vi "LoginGui.vi"(11 "Password":string) -> (3 "ok?":bool)   [LabVIEW 2016]
uses:
  LoginGui.Action.ctl
  tools/Config/Config.Global.vi
panel:
  out "_loop":i32(ring)=4
  in  "pwd_Password":string caption="Password"
  in  "CancelButton":bool
  in  "OKButton":bool
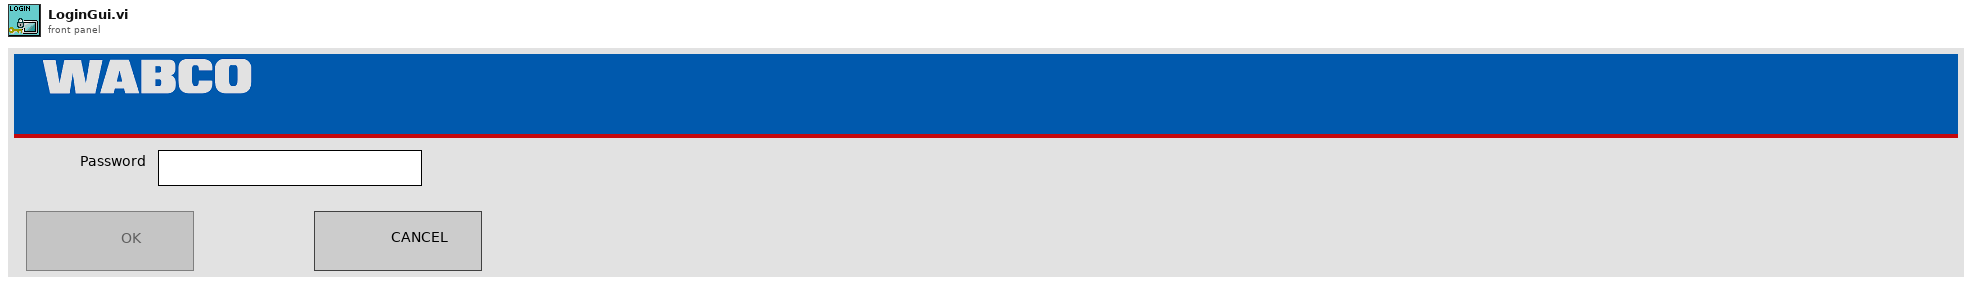
[diagram p1: front panel]
types:
  T1 = typedef "LoginGui.Action.ctl" = enum32{"idle", "constructor", "destructor", "--- Login GUI ---"}
  T2 = enum8{"Enabled", "Disabled", "Disabled and Grayed Out"}
  T3 = enum32{"Invalid", "Default", "Floating", "Floating/Auto-Hide", "Modal"}
  T4 = typedef "FestoCPX.Station.ButtonsState.ctl" = cluster{"Start":bool, "Stop":bool, "Control":bool}
  T5 = typedef "LVPositionTypeDef.ctl" = cluster{"Left":i32, "Top":i32}
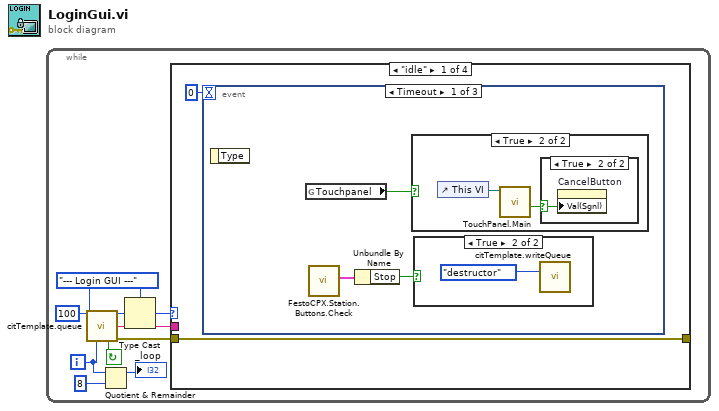
[diagram p0: block diagram]
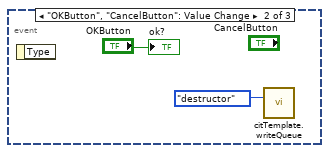
[diagram p5: hidden frame]
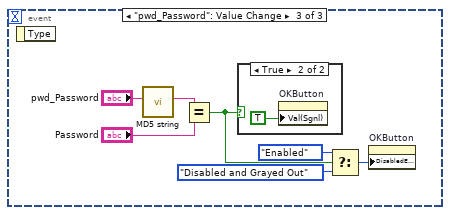
[diagram p6: hidden frame]
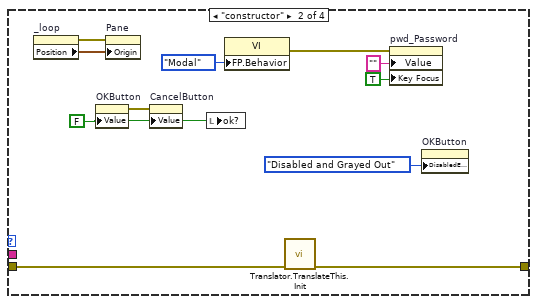
[diagram p8: hidden frame]
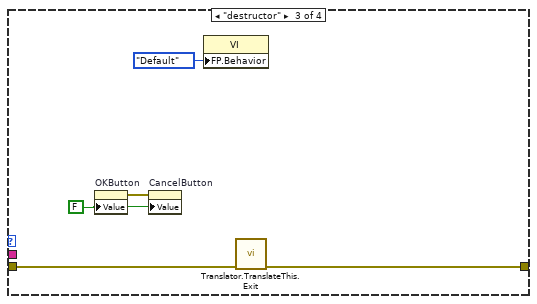
[diagram p9: hidden frame]
diagram:
  n1 = while {
    i -> [w1]
    stop <- w7 continue-if-true
    w6 = LoginGui.Action."--- Login GUI ---" ("Action")
    n2 = call "citTemplate.queue.vi"("ms timeout (250 ms)"=100, "event enum"=w6, "iteration (-1)"=w1) -> ("event out"=w10:u32, "(flatten) data out"=w9:string, "continue"=w7:bool, "error out"=w8:errorcluster)  [unwired: 2 in, 7 out]
    n3 = Quotient & Remainder(x=w1, y=8) -> (x-y*floor(x/y)=→"_loop":i32)  [unwired: 1 out]
    n4 = Type Cast(type=w6, x=w10) -> (*(type *) &x=w5:T1)
    n5 = case shown="\"idle\"" w5 {
      tunnel: w9 -> [_ _ _ _]
      tunnel: w8 -> [w11 w36 w43 w46]
      tunnel: [w11 w35 w42 w46] -> _
      frame "idle" {
        n6 = event shown="[0] Timeout" {
          selector: _ -> [_ _ _]
          dyn-events: _ -> [_ _ _]
          timeout: 0 -> [_ _ _]
          event Timeout {
            n7 = event-data() -> ()  [unwired: 1 in, 1 out]
            n8 = global read "Config.Global.vi" "Touchpanel"() -> (w15:bool)
            n9 = call "FestoCPX.Station.Buttons.Check.vi"() -> ("Buttons.State"=w14:T4)  [unwired: 10 in, 1 out]
            n10 = Unbundle By Name(w14) -> ("Stop"=w13:bool)
            n11 = case shown="True" w15 {
              frame False {
              }
              frame True {
                n12 = control-ref of="This VI"() -> (w18:refnum<vi>)
                n13 = call "TouchPanel.Main.vi"("VI ref"=w18) -> ("Canceled"=w17:bool)  [unwired: 8 in, 2 out]
                n14 = case shown="True" w17 {
                  selector: w17 -> [_ w19]
                  frame False {
                  }
                  frame True {
                    n15 = property on="CancelButton" class="Bool (strict)"("Val(Sgnl)"=w19) -> ()  [unwired: 2 in, 2 out]
                  }
                }
              }
            }
            n16 = case shown="True" w13 {
              frame False {
              }
              frame True {
                n17 = call "citTemplate.writeQueue.vi"("event in (if not connected:all statemachine with data event)"=LoginGui.Action."destructor" ("Action")) -> ()  [unwired: 14 in, 1 out]
              }
            }
          }
          event "OKButton", "CancelButton": Value Change {
            n18 = event-data() -> ()  [unwired: 1 in, 1 out]
            n19 = call "citTemplate.writeQueue.vi"("event in (if not connected:all statemachine with data event)"=LoginGui.Action."destructor" ("Action")) -> ()  [unwired: 14 in, 1 out]
            "ok?" <- "OKButton"
          }
          event "pwd_Password": Value Change {
            n20 = event-data() -> ()  [unwired: 1 in, 1 out]
            n21 = call "MD5 string.vi"("Message String"="pwd_Password") -> ("MD5 message-digest"=w24:string)  [unwired: 10 in]
            n22 = Equal?(x=w24, y="Password") -> (x = y?=w23:bool)
            n23 = case shown="True" w23 {
              frame False {
              }
              frame True {
                n24 = property on="OKButton" class="Bool (strict)"("Val(Sgnl)"=TRUE ("Value (Signaling)")) -> ()  [unwired: 2 in, 2 out]
              }
            }
            n25 = Select(t=T2."Enabled" ("Disabled"), s=w23, f=T2."Disabled and Grayed Out" ("Disabled")) -> (s? t:f=w27:T2)
            n26 = property on="OKButton" class="Bool (strict)"("DisabledEnum"=w27) -> ()  [unwired: 2 in, 2 out]
          }
        }
      }
      frame "constructor" {
        w39 = FALSE ("_b_OK")
        n27 = property on="_loop" class="Ring (strict)"() -> (error out=w37:errorcluster, "Position"=w38:T5)  [unwired: 2 in, 1 out]
        n28 = property on="OKButton" class="Bool (strict)"("Value"=w39) -> (error out=w40:errorcluster)  [unwired: 2 in, 1 out]
        n29 = property on="Pane" class="Pane"(error in=w37, "Origin"=w38) -> ()  [unwired: 1 in, 2 out]
        n30 = property on="CancelButton" class="Bool (strict)"(error in=w40, "Value"=w39) -> ()  [unwired: 1 in, 2 out]
        n31 = local write "ok?"(w39) -> ()
        n32 = property class="VI"("FP.Behavior"=T3."Modal" ("Front Panel Window:Behavior")) -> (error out=w31:errorcluster)  [unwired: 2 in, 1 out]
        n33 = call "Translator.TranslateThis.Init.vi"("error in"=w36) -> ("error out"=w35:errorcluster)  [unwired: 10 in]
        n34 = property on="pwd_Password" class="Str"(error in=w31, "Value"="" ("Password"), "Key Focus"=TRUE) -> ()  [unwired: 1 in, 2 out]
        n35 = property on="OKButton" class="Bool (strict)"("DisabledEnum"=T2."Disabled and Grayed Out" ("Disabled")) -> ()  [unwired: 2 in, 2 out]
      }
      frame "destructor" {
        w44 = FALSE ("_b_OK")
        n36 = property on="OKButton" class="Bool (strict)"("Value"=w44) -> (error out=w45:errorcluster)  [unwired: 2 in, 1 out]
        n37 = property on="CancelButton" class="Bool (strict)"(error in=w45, "Value"=w44) -> ()  [unwired: 1 in, 2 out]
        n38 = property class="VI"("FP.Behavior"=T3."Default" ("Front Panel Window:Behavior")) -> ()  [unwired: 2 in, 2 out]
        n39 = call "Translator.TranslateThis.Exit.vi"("error in"=w43) -> ("error out"=w42:errorcluster)  [unwired: 10 in]
      }
      frame "--- Login GUI ---" {
      }
    }
  }
